vi "test_read-nmea-data2.vi"() -> ()   [LabVIEW 2019] (continued)
53,156,,6*64\n\t\n15:10:38.49\tF9P\t$GPGSV,3,3,09,25,12,307,,6*5A\n\t\n15:10:38.51\tF9P\t$GLGSV,2,1,08,69,12,031,,70,72,041,,71,51,205,19,72,03,209,,1*7A\n\t\n15:10:38.53\tF9P\t$GLGSV,2,2,08,77,01,326,,84,20,122,11,85,70,065,21,86,36,330,,1*78\n\t\n15:10:38.55\tF9P\t$GLGSV,2,1,08,69,12,031,,70,72,041,,71,51,205,17,72,03,209,,3*76\n\t\n15:10:38.57\tF9P\t$GLGSV,2,2,08,77,01,326,,84,20,122,10,85,70,065,21,86,36,330,,3*7B\n\t\n15:10:38.59\tF9P\t$GAGSV,2,1,08,02,09,298,12,04,66,119,31,09,31,193,21,11,71,357,23,7*79\n\t\n15:10:38.61\tF9P\t$GAGSV,2,2,08,12,40,102,08,19,27,045,24,25,09,249,,36,25,308,14,7*70\n\t\n15:10:38.63\tF9P\t$GAGSV,2,1,08,02,09,298,,04,66,119,,09,31,193,,11,71,357,,2*7F\n\t\n15:10:38.65\tF9P\t$GAGSV,2,2,08,12,40,102,,19,27,045,,25,09,249,,36,25,308,,2*7E\n\t\n15:10:38.67\tF9P\t$GBGSV,1,1,03,11,50,131,22,14,87,138,20,33,60,219,20,1*4F\n\t\n15:10:38.69\tF9P\t$GBGSV,1,1,03,11,50,131,26,14,87,138,22,33,60,219,,3*49\n\t\n15:10:38.71\tF9P\t$GNGLL,3723.56308,N,12656.88574,E,061040.00,A,A*79\n\t\n15:10:38.73\tF9P\t\t\n15:10:38.75\tF9P\t\t\n15:10:38.77\tF9P\t\t\n15:10:38.79\tF9P\t\t\n15:10:38.81\tF9P\t\t\n15:10:38.83\tF9P\t\t\n15:10:38.85\tF9P\t\t\n15:10:38.87\tF9P\t\t\n15:10:38.89\tF9P\t\t\n15:10:38.91\tF9P\t\t\n15:10:38.93\tF9P\t\t\n15:10:38.95\tF9P\t\t\n15:10:38.97\tF9P\t\t\n15:10:38.99\tF9P\t\t\n15:10:39.01\tF9P\t\t\n15:10:39.03\tF9P\t\t\n15:10:39.05\tF9P\t\t\n15:10:39.07\tF9P\t\t\n15:10:39.09\tF9P\t\t\n15:10:39.11\tF9P\t\t\n15:10:39.13\tF9P\t\t\n15:10:39.16\tF9P\t\t\n15:10:39.18\tF9P\t\t\n15:10:39.20\tF9P\t\t\n15:10:39.22\tF9P\t\t\n15:10:39.24\tF9P\t$GNRMC,061041.00,A,3723.56224,N,12656.88596,E,2.200,163.36,250720,,,A,V*05\n\t\n15:10:39.26\tF9P\t$GNVTG,163.36,T,,M,2.200,N,4.074,K,A*25\n\t\n15:10:39.28\tF9P\t$GNGGA,061041.00,3723.56224,N,12656.88596,E,1,12,0.64,65.3,M,18.5,M,,*73\n\t\n15:10:39.30\tF9P\t$GNGSA,A,3,12,06,19,05,17,09,04,02,,,,,1.18,0.64,1.00,1*0B\n\t\n15:10:39.32\tF9P\t$GNGSA,A,3,85,71,84,,,,,,,,,,1.18,0.64,1.00,2*0E\n\t\n15:10:39.34\tF9P\t$GNGSA,A,3,36,19,11,04,09,12,,,,,,,1.18,0.64,1.00,3*0B\n\t\n15:10:39.36\tF9P\t$GNGSA,A,3,14,11,33,,,,,,,,,,1.18,0.64,1.00,4*0A\n\t\n15:10:39.38\tF9P\t$GPGSV,3,1,09,02,54,318,25,04,18,044,23,05,37,247,27,06,64,047,33,1*6F\n\t\n15:10:39.40\tF9P\t$GPGSV,3,2,09,09,45,074,22,12,24,277,24,17,34,153,25,19,53,156,30,1*68\n\t\n15:10:39.42\tF9P\t$GPGSV,3,3,09,25,12,307,20,1*5F\n\t\n15:10:39.44\tF9P\t$GPGSV,3,1,09,02,54,318,,04,18,044,,05,37,247,,06,64,047,16,6*6C\n\t\n15:10:39.46\tF9P\t$GPGSV,3,2,09,09,45,074,,12,24,277,,17,34,153,19,19,53,156,,6*65\n\t\n15:10:39.48\tF9P\t$GPGSV,3,3,09,25,12,307,,6*5A\n\t\n15:10:39.50\tF9P\t$GLGSV,2,1,08,69,12,031,,70,72,041,,71,51,205,20,72,03,209,,1*70\n\t\n15:10:39.52\tF9P\t$GLGSV,2,2,08,77,01,326,,84,20,122,11,85,70,065,23,86,36,330,,1*7A\n\t\n15:10:39.54\tF9P\t$GLGSV,2,1,08,69,12,031,,70,72,041,,71,51,205,17,72,03,209,,3*76\n\t\n15:10:39.56\tF9P\t$GLGSV,2,2,08,77,01,326,,84,20,122,11,85,70,065,20,86,36,330,,3*7B\n\t\n15:10:39.58\tF9P\t$GAGSV,2,1,08,02,09,298,10,04,66,119,29,09,31,193,22,11,71,357,22,7*70\n\t\n15:10:39.60\tF9P\t$GAGSV,2,2,08,12,40,102,15,19,27,045,22,25,09,249,,36,25,308,17,7*79\n\t\n15:10:39.62\tF9P\t$GAGSV,2,1,08,02,09,298,,04,66,119,,09,31,193,,11,71,357,,2*7F\n\t\n15:10:39.64\tF9P\t$GAGSV,2,2,08,12,40,102,,19,27,045,,25,09,249,,36,25,308,,2*7E\n\t\n15:10:39.66\tF9P\t$GBGSV,1,1,03,11,50,131,22,14,87,138,21,33,60,219,21,1*4F\n\t\n15:10:39.68\tF9P\t$GBGSV,1,1,03,11,50,131,26,14,87,138,21,33,60,219,,3*4A\n\t\n15:10:39.70\tF9P\t$GNGLL,3723.56224,N,12656.88596,E,061041.00,A,A*7B\n\t\n15:10:39.72\tF9P\t\t\n15:10:39.74\tF9P\t\t\n15:10:39.76\tF9P\t\t\n15:10:39.78\tF9P\t\t\n15:10:39.80\tF9P\t\t\n15:10:39.82\tF9P\t\t\n15:10:39.84\tF9P\t\t\n15:10:39.86\tF9P\t\t\n15:10:39.88\tF9P\t\t\n15:10:39.90\tF9P\t\t\n15:10:39.92\tF9P\t\t\n15:10:39.94\tF9P\t\t\n15:10:39.96\tF9P\t\t\n15:10:39.98\tF9P\t\t\n15:10:40.00\tF9P\t\t\n15:10:40.02\tF9P\t\t\n15:10:40.04\tF9P\t\t\n15:10:40.06\tF9P\t\t\n15:10:40.08\tF9P\t\t\n15:10:40.10\tF9P\t\t\n15:10:40.12\tF9P\t\t\n15:10:40.14\tF9P\t\t\n15:10:40.16\tF9P\t\t\n15:10:40.18\tF9P\t\t\n15:10:40.20\tF9P\t\t\n15:10:40.22\tF9P\t\t\n15:10:40.24\tF9P\t\t\n15:10:40.26\tF9P\t$GNRMC,061042.00,A,3723.56162,N,12656.88593,E,1.234,,250720,,,A,V*19\n\t\n15:10:40.28\tF9P\t$GNVTG,,T,,M,1.234,N,2.285,K,A*34\n\t\n15:10:40.30\tF9P\t$GNGGA,061042.00,3723.56162,N,12656.88593,E,1,12,0.64,65.2,M,18.5,M,,*75\n\t\n15:10:40.32\tF9P\t$GNGSA,A,3,12,06,19,05,17,09,04,02,,,,,1.18,0.64,1.00,1*0B\n\t\n15:10:40.34\tF9P\t$GNGSA,A,3,85,71,84,,,,,,,,,,1.18,0.64,1.00,2*0E\n\t\n15:10:40.36\tF9P\t$GNGSA,A,3,36,19,11,04,09,12,,,,,,,1.18,0.64,1.00,3*0B\n\t\n15:10:40.38\tF9P\t$GNGSA,A,3,14,11,33,,,,,,,,,,1.18,0.64,1.00,4*0A\n\t\n15:10:40.40\tF9P\t$GPGSV,3,1,09,02,54,318,26,04,18,044,25,05,37,247,27,06,64,047,34,1*6D\n\t\n15:10:40.42\tF9P\t$GPGSV,3,2,09,09,45,074,22,12,24,277,24,17,33,153,26,19,53,156,23,1*6E\n\t\n15:10:40.44\tF9P\t$GPGSV,3,3,09,25,12,307,27,1*58\n\t\n15:10:40.46\tF9P\t$GPGSV,3,1,09,02,54,318,,04,18,044,,05,37,247,,06,64,047,16,6*6C\n\t\n15:10:40.48\tF9P\t$GPGSV,3,2,09,09,45,074,,12,24,277,,17,33,153,21,19,53,156,,6*69\n\t\n15:10:40.50\tF9P\t$GPGSV,3,3,09,25,12,307,27,6*5F\n\t\n15:10:40.52\tF9P\t$GLGSV,2,1,08,69,12,031,,70,72,041,,71,51,205,20,72,03,209,,1*70\n\t\n15:10:40.54\tF9P\t$GLGSV,2,2,08,77,01,326,,84,20,122,09,85,70,065,22,86,36,330,,1*72\n\t\n15:10:40.56\tF9P\t$GLGSV,2,1,08,69,12,031,,70,72,041,,71,51,205,19,72,03,209,,3*78\n\t\n15:10:40.58\tF9P\t$GLGSV,2,2,08,77,01,326,,84,20,122,08,85,70,065,20,86,36,330,,3*73\n\t\n15:10:40.60\tF9P\t$GAGSV,2,1,08,02,09,298,10,04,66,119,28,09,31,193,24,11,71,357,22,7*77\n\t\n15:10:40.62\tF9P\t$GAGSV,2,2,08,12,40,102,10,19,27,045,20,25,09,249,,36,25,308,17,7*7E\n\t\n15:10:40.64\tF9P\t$GAGSV,2,1,08,02,09,298,,04,66,119,,09,31,193,,11,71,357,,2*7F\n\t\n15:10:40.66\tF9P\t$GAGSV,2,2,08,12,40,102,,19,27,045,,25,09,249,,36,25,308,,2*7E\n\t\n15:10:40.68\tF9P\t$GBGSV,1,1,03,11,50,131,22,14,87,138,20,33,60,219,20,1*4F\n\t\n15:10:40.70\tF9P\t$GBGSV,1,1,03,11,50,131,,14,87,138,21,33,60,219,,3*4E\n\t\n15:10:40.72\tF9P\t$GNGLL,3723.56162,N,12656.88593,E,061042.00,A,A*7C\n\t\n15:10:40.74\tF9P\t\t\n15:10:40.76\tF9P\t\t\n15:10:40.78\tF9P\t\t\n15:10:40.80\tF9P\t\t\n15:10:40.82\tF9P\t\t\n15:10:40.84\tF9P\t\t\n15:10:40.86\tF9P\t\t\n15:10:40.88\tF9P\t\t\n15:10:40.90\tF9P\t\t\n15:10:40.92\tF9P\t\t\n15:10:40.94\tF9P\t\t\n15:10:40.96\tF9P\t\t\n15:10:40.98\tF9P\t\t\n15:10:41.00\tF9P\t\t\n15:10:41.02\tF9P\t\t\n15:10:41.04\tF9P\t\t\n15:10:41.06\tF9P\t\t\n15:10:41.08\tF9P\t\t\n15:10:41.10\tF9P\t\t\n15:10:41.12\tF9P\t\t\n15:10:41.14\tF9P\t\t\n15:10:41.16\tF9P\t\t\n15:10:41.18\tF9P\t\t\n15:10:41.20\tF9P\t\t\n15:10:41.22\tF9P\t\t\n15:10:41.24\tF9P\t$GNRMC,061043.00,A,3723.56127,N,12656.88611,E,0.413,,250720,,,A,V*12\n\t\n15:10:41.26\tF9P\t$GNVTG,,T,,M,0.413,N,0.766,K,A*3C\n\t\n15:10:41.28\tF9P\t$GNGGA,061043.00,3723.56127,N,12656.88611,E,1,12,0.70,65.9,M,18.5,M,,*72\n\t\n15:10:41.30\tF9P\t$GNGSA,A,3,12,06,19,05,17,09,04,02,,,,,1.25,0.70,1.03,1*03\n\t\n15:10:41.32\tF9P\t$GNGSA,A,3,85,71,84,,,,,,,,,,1.25,0.70,1.03,2*06\n\t\n15:10:41.34\tF9P\t$GNGSA,A,3,36,19,11,04,09,12,,,,,,,1.25,0.70,1.03,3*03\n\t\n15:10:41.36\tF9P\t$GNGSA,A,3,14,11,33,,,,,,,,,,1.25,0.70,1.03,4*02\n\t\n15:10:41.38\tF9P\t$GPGSV,3,1,09,02,54,318,26,04,18,044,24,05,37,247,25,06,64,047,30,1*6A\n\t\n15:10:41.40\tF9P\t$GPGSV,3,2,09,09,45,074,21,12,24,277,24,17,33,153,26,19,53,156,29,1*67\n\t\n15:10:41.42\tF9P\t$GPGSV,3,3,09,25,12,307,26,1*59\n\t\n15:10:41.44\tF9P\t$GPGSV,3,1,09,02,54,318,,04,18,044,17,05,37,247,,06,64,047,15,6*69\n\t\n15:10:41.46\tF9P\t$GPGSV,3,2,09,09,45,074,,12,24,277,,17,33,153,20,19,53,156,,6*68\n\t\n15:10:41.48\tF9P\t$GPGSV,3,3,09,25,12,307,23,6*5B\n\t\n15:10:41.50\tF9P\t$GLGSV,2,1,08,69,12,031,,70,72,041,,71,51,205,20,72,03,209,,1*70\n\t\n15:10:41.52\tF9P\t$GLGSV,2,2,08,77,01,326,,84,20,122,09,85,70,065,21,86,36,330,,1*71\n\t\n15:10:41.54\tF9P\t$GLGSV,2,1,08,69,12,031,,70,72,041,,71,51,205,19,72,03,209,,3*78\n\t\n15:10:41.56\tF9P\t$GLGSV,2,2,08,77,01,326,,84,20,122,12,85,70,065,20,86,36,330,,3*78\n\t\n15:10:41.58\tF9P\t$GAGSV,2,1,08,02,09,298,10,04,66,119,28,09,31,193,23,11,71,357,22,7*70\n\t\n15:10:41.60\tF9P\t$GAGSV,2,2,08,12,40,102,14,19,27,045,19,25,09,249,,36,25,308,11,7*76\n\t\n15:10:41.62\tF9P\t$GAGSV,2,1,08,02,09,298,,04,66,119,,09,31,193,,11,71,357,,2*7F\n\t\n15:10:41.64\tF9P\t$GAGSV,2,2,08,12,40,102,,19,27,045,,25,09,249,,36,25,308,,2*7E\n\t\n15:10:41.66\tF9P\t$GBGSV,1,1,03,11,50,131,21,14,87,138,21,33,60,219,19,1*47\n\t\n15:10:41.68\tF9P\t$GBGSV,1,1,03,11,50,131,,14,87,138,,33,60,219,,3*4D\n\t\n15:10:41.70\tF9P\t$GNGLL,3723.56127,N,12656.88611,E,061043.00,A,A*75\n\t\n15:10:41.72\tF9P\t\t\n15:10:41.74\tF9P\t\t\n15:10:41.76\tF9P\t\t\n15:10:41.78\tF9P\t\t\n15:10:41.80\tF9P\t\t\n15:10:41.82\tF9P\t\t\n15:10:41.84\tF9P\t\t\n15:10:41.86\tF9P\t\t\n15:10:41.88\tF9P\t\t\n15:10:41.90\tF9P\t\t\n15:10:41.92\tF9P\t\t\n15:10:41.94\tF9P\t\t\n15:10:41.96\tF9P\t\t\n15:10:41.98\tF9P\t\t\n15:10:42.00\tF9P\t\t\n15:10:42.02\tF9P\t\t\n15:10:42.04\tF9P\t\t\n15:10:42.06\tF9P\t\t\n15:10:42.08\tF9P\t\t\n15:10:42.10\tF9P\t\t\n15:10:42.12\tF9P\t\t\n15:10:42.14\tF9P\t\t\n15:10:42.16\tF9P\t\t\n15:10:42.18\tF9P\t\t\n15:10:42.20\tF9P\t\t\n15:10:42.22\tF9P\t\t\n15:10:42.24\tF9P\t\t\n15:10:42.26\tF9P\t$GNRMC,061044.00,A,3723.56052,N,12656.88629,E,1.835,,250720,,,A,V*14\n\t\n15:10:42.28\tF9P\t$GNVTG,,T,,M,1.835,N,3.398,K,A*33\n\t\n15:10:42.30\tF9P\t$GNGGA,061044.00,3723.56052,N,12656.88629,E,1,12,0.64,65.7,M,18.5,M,,*76\n\t\n15:10:42.32\tF9P\t$GNGSA,A,3,12,06,19,05,17,09,04,02,,,,,1.18,0.64,1.00,1*0B\n\t\n15:10:42.34\tF9P\t$GNGSA,A,3,85,71,84,,,,,,,,,,1.18,0.64,1.00,2*0E\n\t\n15:10:42.36\tF9P\t$GNGSA,A,3,36,19,11,04,09,12,,,,,,,1.18,0.64,1.00,3*0B\n\t\n15:10:42.38\tF9P\t$GNGSA,A,3,14,11,33,,,,,,,,,,1.18,0.64,1.00,4*0A\n\t\n15:10:42.40\tF9P\t$GPGSV,3,1,09,02,54,318,27,04,18,044,22,05,37,247,24,06,64,047,22,1*6F\n\t\n15:10:42.42\tF9P\t$GPGSV,3,2,09,09,45,074,21,12,24,277,22,17,33,153,27,19,53,157,29,1*61\n\t\n15:10:42.44\tF9P\t$GPGSV,3,3,09,25,12,307,26,1*59\n\t\n15:10:42.46\tF9P\t$GPGSV,3,1,09,02,54,318,,04,18,044,,05,37,247,18,06,64,047,16,6*65\n\t\n15:10:42.48\tF9P\t$GPGSV,3,2,09,09,45,074,,12,24,277,,17,33,153,19,19,53,157,,6*63\n\t\n15:10:42.50\tF9P\t$GPGSV,3,3,09,25,12,307,20,6*58\n\t\n15:10:42.52\tF9P\t$GLGSV,2,1,08,69,12,031,,70,72,041,,71,51,205,20,72,03,209,,1*70\n\t\n15:10:42.54\tF9P\t$GLGSV,2,2,08,77,01,326,,84,20,122,08,85,70,065,24,86,36,330,,1*75\n\t\n15:10:42.56\tF9P\t$GLGSV,2,1,08,69,12,031,,70,72,041,,71,51,205,22,72,03,209,,3*70\n\t\n15:10:42.58\tF9P\t$GLGSV,2,2,08,77,01,326,,84,20,122,11,85,70,065,21,86,36,330,,3*7A\n\t\n15:10:42.60\tF9P\t$GAGSV,2,1,08,02,09,298,11,04,66,119,26,09,31,193,21,11,71,357,21,7*7E\n\t\n15:10:42.62\tF9P\t$GAGSV,2,2,08,12,40,102,17,19,27,045,16,25,09,249,,36,25,308,13,7*78\n\t\n15:10:42.64\tF9P\t$GAGSV,2,1,08,02,09,298,,04,66,119,,09,31,193,,11,71,357,,2*7F\n\t\n15:10:42.66\tF9P\t$GAGSV,2,2,08,12,40,102,,19,27,045,,25,09,249,,36,25,308,,2*7E\n\t\n15:10:42.68\tF9P\t$GBGSV,1,1,03,11,50,131,22,14,87,138,21,33,60,219,19,1*44\n\t\n15:10:42.70\tF9P\t$GBGSV,1,1,03,11,50,131,,14,87,138,,33,60,219,,3*4D\n\t\n15:10:42.72\tF9P\t$GNGLL,3723.56052,N,12656.88629,E,061044.00,A,A*7A\n\t\n15:10:42.74\tF9P\t\t\n15:10:42.76\tF9P\t\t\n15:10:42.78\tF9P\t\t\n15:10:42.80\tF9P\t\t\n15:10:42.82\tF9P\t\t\n15:10:42.84\tF9P\t\t\n15:10:42.86\tF9P\t\t\n15:10:42.88\tF9P\t\t\n15:10:42.90\tF9P\t\t\n15:10:42.92\tF9P\t\t\n15:10:42.94\tF9P\t\t\n15:10:42.96\tF9P\t\t\n15:10:42.98\tF9P\t\t\n15:10:43.00\tF9P\t\t\n15:10:43.02\tF9P\t\t\n15:10:43.04\tF9P\t\t\n15:10:43.06\tF9P\t\t\n15:10:43.08\tF9P\t\t\n15:10:43.10\tF9P\t\t\n15:10:43.12\tF9P\t\t\n15:10:43.14\tF9P\t\t\n15:10:43.16\tF9P\t\t\n15:10:43.18\tF9P\t\t\n15:10:43.20\tF9P\t\t\n15:10:43.22\tF9P\t\t\n15:10:43.24\tF9P\t$GNRMC,061045.00,A,3723.55971,N,12656.88668,E,1.690,,250720,,,A,V*1A\n\t\n15:10:43.26\tF9P\t$GNVTG,,T,,M,1.690,N,3.129,K,A*3A\n\t\n15:10:43.28\tF9P\t$GNGGA,061045.00,3723.55971,N,12656.88668,E,1,12,0.64,65.2,M,18.5,M,,*7C\n\t\n15:10:43.30\tF9P\t$GNGSA,A,3,12,06,19,05,17,09,04,02,,,,,1.18,0.64,1.00,1*0B\n\t\n15:10:43.32\tF9P\t$GNGSA,A,3,85,71,84,,,,,,,,,,1.18,0.64,1.00,2*0E\n\t\n15:10:43.34\tF9P\t$GNGSA,A,3,36,19,11,04,09,12,,,,,,,1.18,0.64,1.00,3*0B\n\t\n15:10:43.36\tF9P\t$GNGSA,A,3,14,11,33,,,,,,,,,,1.18,0.64,1.00,4*0A\n\t\n15:10:43.38\tF9P\t$GPGSV,3,1,09,02,54,318,26,04,18,044,20,05,37,247,23,06,64,047,19,1*63\n\t\n15:10:43.40\tF9P\t$GPGSV,3,2,09,09,45,074,19,12,24,277,22,17,33,153,32,19,53,157,19,1*6D\n\t\n15:10:43.42\tF9P\t$GPGSV,3,3,09,25,12,307,22,1*5D\n\t\n15:10:43.44\tF9P\t$GPGSV,3,1,09,02,54,318,,04,18,044,,05,37,247,16,06,64,047,17,6*6A\n\t\n15:10:43.46\tF9P\t$GPGSV,3,2,09,09,45,074,,12,24,277,,17,33,153,18,19,53,157,,6*62\n\t\n15:10:43.48\tF9P\t$GPGSV,3,3,09,25,12,307,20,6*58\n\t\n15:10:43.50\tF9P\t$GLGSV,2,1,08,69,12,031,,70,72,041,,71,51,205,20,72,03,209,,1*70\n\t\n15:10:43.52\tF9P\t$GLGSV,2,2,08,77,01,326,,84,20,122,08,85,70,065,23,86,36,330,,1*72\n\t\n15:10:43.54\tF9P\t$GLGSV,2,1,08,69,12,031,,70,72,041,,71,51,205,23,72,03,209,,3*71\n\t\n15:10:43.56\tF9P\t$GLGSV,2,2,08,77,01,326,,84,20,122,08,85,70,065,21,86,36,330,,3*72\n\t\n15:10:43.58\tF9P\t$GAGSV,2,1,08,02,09,298,10,04,66,119,24,09,31,193,20,11,71,357,20,7*7D\n\t\n15:10:43.60\tF9P\t$GAGSV,2,2,08,12,40,102,10,19,27,045,14,25,09,249,,36,25,308,11,7*7F\n\t\n15:10:43.62\tF9P\t$GAGSV,2,1,08,02,09,298,,04,66,119,,09,31,193,,11,71,357,,2*7F\n\t\n15:10:43.64\tF9P\t$GAGSV,2,2,08,12,40,102,,19,27,045,,25,09,249,,36,25,308,,2*7E\n\t\n15:10:43.66\tF9P\t$GBGSV,1,1,03,11,50,131,21,14,87,138,21,33,60,219,18,1*46\n\t\n15:10:43.68\tF9P\t$GBGSV,1,1,03,11,50,131,30,14,87,138,,33,60,219,,3*4E\n\t\n15:10:43.70\tF9P\t$GNGLL,3723.55971,N,12656.88668,E,061045.00,A,A*75\n\t\n15:10:43.72\tF9P\t\t\n15:10:43.74\tF9P\t\t\n15:10:43.76\tF9P\t\t\n15:10:43.78\tF9P\t\t\n15:10:43.80\tF9P\t\t\n15:10:43.82\tF9P\t\t\n15:10:43.84\tF9P\t\t\n15:10:43.86\tF9P\t\t\n15:10:43.88\tF9P\t\t\n15:10:43.90\tF9P\t\t\n15:10:43.92\tF9P\t\t\n15:10:43.94\tF9P\t\t\n15:10:43.96\tF9P\t\t\n15:10:43.98\tF9P\t\t\n15:10:44.00\tF9P\t\t\n15:10:44.02\tF9P\t\t\n15:10:44.04\tF9P\t\t\n15:10:44.06\tF9P\t\t\n15:10:44.08\tF9P\t\t\n15:10:44.10\tF9P\t\t\n15:10:44.12\tF9P\t\t\n15:10:44.14\tF9P\t\t\n15:10:44.16\tF9P\t\t\n15:10:44.18\tF9P\t\t\n15:10:44.20\tF9P\t\t\n15:10:44.22\tF9P\t\t\n15:10:44.24\tF9P\t$GNRMC,061046.00,A,3723.55907,N,12656.88711,E,1.906,,250720,,,A,V*17\n\t\n15:10:44.26\tF9P\t$GNVTG,,T,,M,1.906,N,3.530,K,A*36\n\t\n15:10:44.28\tF9P\t$GNGGA,061046.00,3723.55907,N,12656.88711,E,1,12,0.64,64.9,M,18.5,M,,*7B\n\t\n15:10:44.30\tF9P\t$GNGSA,A,3,12,06,19,05,17,09,04,02,,,,,1.18,0.64,1.00,1*0B\n\t\n15:10:44.32\tF9P\t$GNGSA,A,3,85,71,84,,,,,,,,,,1.18,0.64,1.00,2*0E\n\t\n15:10:44.34\tF9P\t$GNGSA,A,3,36,19,11,04,09,12,,,,,,,1.18,0.64,1.00,3*0B\n\t\n15:10:44.36\tF9P\t$GNGSA,A,3,14,11,33,,,,,,,,,,1.18,0.64,1.00,4*0A\n\t\n15:10:44.38\tF9P\t$GPGSV,3,1,09,02,54,318,26,04,18,044,18,05,37,247,22,06,64,047,30,1*62\n\t\n15:10:44.40\tF9P\t$GPGSV,3,2,09,09,45,074,19,12,24,277,22,17,33,153,27,19,53,157,21,1*62\n\t\n15:10:44.42\tF9P\t$GPGSV,3,3,09,25,12,307,20,1*5F\n\t\n15:10:44.44\tF9P\t$GPGSV,3,1,09,02,54,318,,04,18,044,,05,37,247,11,06,64,047,16,6*6C\n\t\n15:10:44.46\tF9P\t$GPGSV,3,2,09,09,45,074,,12,24,277,,17,33,153,17,19,53,157,,6*6D\n\t\n15:10:44.48\tF9P\t$GPGSV,3,3,09,25,12,307,16,6*5D\n\t\n15:10:44.50\tF9P\t$GLGSV,2,1,08,69,12,031,,70,72,041,,71,51,205,19,72,03,209,,1*7A\n\t\n15:10:44.52\tF9P\t$GLGSV,2,2,08,77,01,326,,84,20,122,10,85,70,065,23,86,36,330,,1*7B\n\t\n15:10:44.54\tF9P\t$GLGSV,2,1,08,69,12,031,,70,72,041,,71,51,205,22,72,03,209,,3*70\n\t\n15:10:44.56\tF9P\t$GLGSV,2,2,08,77,01,326,,84,20,122,12,85,70,065,20,86,36,330,,3*78\n\t\n15:10:44.58\tF9P\t$GAGSV,2,1,08,02,09,298,09,04,66,119,27,09,31,193,22,11,71,357,22,7*76\n\t\n15:10:44.60\tF9P\t$GAGSV,2,2,08,12,40,102,19,19,27,045,16,25,09,249,,36,25,308,10,7*75\n\t\n15:10:44.62\tF9P\t$GAGSV,2,1,08,02,09,298,,04,66,119,,09,31,193,,11,71,357,,2*7F\n\t\n15:10:44.64\tF9P\t$GAGSV,2,2,08,12,40,102,,19,27,045,,25,09,249,,36,25,308,,2*7E\n\t\n15:10:44.66\tF9P\t$GBGSV,1,1,03,11,50,131,21,14,87,138,23,33,60,219,21,1*4E\n\t\n15:10:44.68\tF9P\t$GBGSV,1,1,03,11,50,131,,14,87,138,,33,60,219,,3*4D\n\t\n15:10:44.70\tF9P\t$GNGLL,3723.55907,N,12656.88711,E,061046.00,A,A*78\n\t\n15:10:44.72\tF9P\t\t\n15:10:44.74\tF9P\t\t\n15:10:44.76\tF9P\t\t\n15:10:44.78\tF9P\t\t\n15:10:44.80\tF9P\t\t\n15:10:44.82\tF9P\t\t\n15:10:44.84\tF9P\t\t\n15:10:44.86\tF9P\t\t\n15:10:44.88\tF9P\t\t\n15:10:44.90\tF9P\t\t\n15:10:44.92\tF9P\t\t\n15:10:44.94\tF9P\t\t\n15:10:44.96\tF9P\t\t\n15:10:44.98\tF9P\t\t\n15:10:45.00\tF9P\t\t\n15:10:45.02\tF9P\t\t\n15:10:45.04\tF9P\t\t\n15:10:45.06\tF9P\t\t\n15:10:45.08\tF9P\t\t\n15:10:45.10\tF9P\t\t\n15:10:45.12\tF9P\t\t\n15:10:45.14\tF9P\t\t\n15:10:45.16\tF9P\t\t\n15:10:45.18\tF9P\t\t\n15:10:45.20\tF9P\t\t\n15:10:45.22\tF9P\t\t\n15:10:45.24\tF9P\t$GNRMC,061047.00,A,3723.55836,N,12656.88735,E,2.335,,250720,,,A,V*1A\n\t\n15:10:45.26\tF9P\t$GNVTG,,T,,M,2.335,N,4.325,K,A*3A\n\t\n15:10:45.28\tF9P\t$GNGGA,061047.00,3723.55836,N,12656.88735,E,1,12,0.64,64.8,M,18.5,M,,*7E\n\t\n15:10:45.30\tF9P\t$GNGSA,A,3,12,06,19,05,17,09,04,02,,,,,1.18,0.64,1.00,1*0B\n\t\n15:10:45.32\tF9P\t$GNGSA,A,3,85,71,84,,,,,,,,,,1.18,0.64,1.00,2*0E\n\t\n15:10:45.34\tF9P\t$GNGSA,A,3,36,19,11,04,09,12,,,,,,,1.18,0.64,1.00,3*0B\n\t\n15:10:45.36\tF9P\t$GNGSA,A,3,14,11,33,,,,,,,,,,1.18,0.64,1.00,4*0A\n\t\n15:10:45.38\tF9P\t$GPGSV,3,1,09,02,54,318,31,04,18,044,18,05,37,247,21,06,64,047,25,1*63\n\t\n15:10:45.40\tF9P\t$GPGSV,3,2,09,09,45,074,18,12,24,277,22,17,33,153,26,19,53,157,22,1*61\n\t\n15:10:45.42\tF9P\t$GPGSV,3,3,09,25,12,307,19,1*55\n\t\n15:10:45.44\tF9P\t$GPGSV,3,1,09,02,54,318,,04,18,044,,05,37,247,08,06,64,047,15,6*67\n\t\n15:10:45.46\tF9P\t$GPGSV,3,2,09,09,45,074,,12,24,277,,17,33,153,17,19,53,157,,6*6D\n\t\n15:10:45.48\tF9P\t$GPGSV,3,3,09,25,12,307,14,6*5F\n\t\n15:10:45.50\tF9P\t$GLGSV,2,1,08,69,12,031,,70,72,041,,71,51,205,19,72,03,209,,1*7A\n\t\n15:10:45.52\tF9P\t$GLGSV,2,2,08,77,01,326,,84,20,122,09,85,70,065,22,86,36,330,,1*72\n\t\n15:10:45.54\tF9P\t$GLGSV,2,1,08,69,12,031,,70,72,041,,71,51,205,23,72,03,209,,3*71\n\t\n15:10:45.56\tF9P\t$GLGSV,2,2,08,77,01,326,,84,20,122,13,85,70,065,19,86,36,330,,3*73\n\t\n15:10:45.58\tF9P\t$GAGSV,2,1,08,02,09,298,10,04,66,119,24,09,31,193,22,11,71,357,22,7*7D\n\t\n15:10:45.60\tF9P\t$GAGSV,2,2,08,12,40,102,15,19,27,045,15,25,09,249,,36,25,308,15,7*7F\n\t\n15:10:45.62\tF9P\t$GAGSV,2,1,08,02,09,298,,04,66,119,,09,31,193,,11,71,357,,2*7F\n\t\n15:10:45.64\tF9P\t$GAGSV,2,2,08,12,40,102,,19,27,045,,25,09,249,,36,25,308,,2*7E\n\t\n15:10:45.66\tF9P\t$GBGSV,1,1,03,11,50,131,20,14,87,138,21,33,60,219,21,1*4D\n\t\n15:10:45.68\tF9P\t$GBGSV,1,1,03,11,50,131,31,14,87,138,,33,60,219,,3*4F\n\t\n15:10:45.70\tF9P\t$GNGLL,3723.55836,N,12656.88735,E,061047.00,A,A*7C\n\t\n15:10:45.72\tF9P\t\t\n15:10:45.74\tF9P\t\t\n15:10:45.76\tF9P\t\t\n15:10:45.78\tF9P\t\t\n15:10:45.80\tF9P\t\t\n15:10:45.82\tF9P\t\t\n15:10:45.84\tF9P\t\t\n15:10:45.86\tF9P\t\t\n15:10:45.88\tF9P\t\t\n15:10:45.90\tF9P\t\t\n15:10:45.92\tF9P\t\t\n15:10:45.94\tF9P\t\t\n15:10:45.96\tF9P\t\t\n15:10:45.98\tF9P\t\t\n15:10:46.00\tF9P\t\t\n15:10:46.02\tF9P\t\t\n15:10:46.04\tF9P\t\t\n15:10:46.06\tF9P\t\t\n15:10:46.08\tF9P\t\t\n15:10:46.10\tF9P\t\t\n15:10:46.12\tF9P\t\t\n15:10:46.14\tF9P\t\t\n15:10:46.16\tF9P\t\t\n15:10:46.18\tF9P\t\t\n15:10:46.20\tF9P\t\t\n15:10:46.22\tF9P\t\t\n15:10:46.24\tF9P\t$GNRMC,061048.00,A,3723.55761,N,12656.88740,E,2.445,166.66,250720,,,A,V*05\n\t\n15:10:46.26\tF9P\t$GNVTG,166.66,T,,M,2.445,N,4.528,K,A*2E\n\t\n15:10:46.28\tF9P\t$GNGGA,061048.00,3723.55761,N,12656.88740,E,1,12,0.64,65.2,M,18.5,M,,*75\n\t\n15:10:46.30\tF9P\t$GNGSA,A,3,12,06,19,05,17,09,04,02,,,,,1.18,0.64,1.00,1*0B\n\t\n15:10:46.32\tF9P\t$GNGSA,A,3,85,71,84,,,,,,,,,,1.18,0.64,1.00,2*0E\n\t\n15:10:46.34\tF9P\t$GNGSA,A,3,36,19,11,04,09,12,,,,,,,1.18,0.64,1.00,3*0B\n\t\n15:10:46.36\tF9P\t$GNGSA,A,3,14,11,33,,,,,,,,,,1.18,0.64,1.00,4*0A\n\t\n15:10:46.38\tF9P\t$GPGSV,3,1,09,02,54,318,33,04,18,044,16,05,37,247
